vi "Add Property.vi"(6 "String?":bool, 7 "Include Empty?":bool, 9 "Value":string, 10 "Property Name":string, 11 "String In":string="{") -> (3 "String out":string)   [LabVIEW 2015, in "JSON.lvlib"]
doc: "This VI does not generate complete JSON!\n\nThis is a utility VI to help build partial JSON strings by adding a property to an object. If the property added isn't the first added to an object (the preceding character isn't '{') then it will prepend the property with the necessary comma. For this to work properly the first item being added should have \"{\" passed in as the partial JSON string and after all properties are added the JSON must be closed with \"}\"."
uses:
  JSON.lvlib
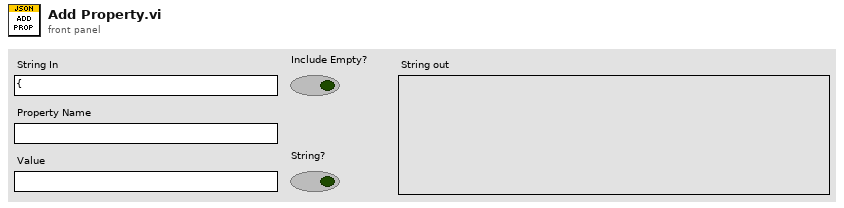
[diagram p1: front panel]
types:
  T1 = typedef "JSON.lvlib/JSON Item Type.ctl" = enum16{"unknown", "null", "Array", "Object", "String", "Number", "Boolean"}
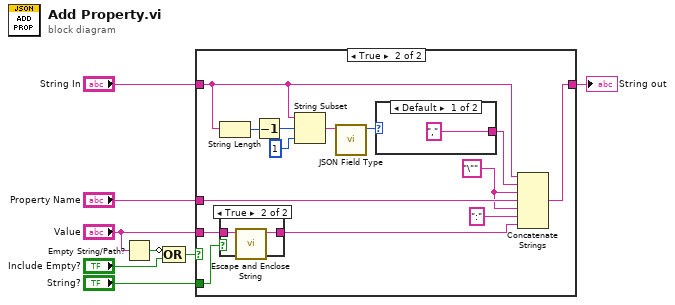
[diagram p0: block diagram]
diagram:
  n1 = Empty String/Path?(string/path="Value") -> (empty?=w8:bool)
  n2 = Compound Arithmetic op=OR(invert w8, "Include Empty?") -> (w6:bool)
  n3 = case shown="True" w6 {
    tunnel: "Value" -> [_ w19]
    tunnel: "Property Name" -> [_ w14]
    tunnel: "String In" -> [w9 w16]
    tunnel: [w9 w10] -> w2
    tunnel: "String?" -> [_ w18]
    frame False {
    }
    frame True {
      w11 = "\"" ("string")
      n4 = String Length(string=w16) -> (length=w23:i32)
      n5 = case shown="True" w18 {
        tunnel: w19 -> [w25 w27]
        tunnel: [w25 w26] -> w12
        frame False {
        }
        frame True {
          n6 = call "Escape and Enclose String.vi"("String"=w27) -> ("JSON String"=w26:string)  [unwired: 10 in]
        }
      }
      n7 = Decrement(x=w23) -> (x-1=w22:i32)
      n8 = String Subset(string=w16, offset (0)=w22, length (rest)=1 ("length (rest)")) -> (substring=w20:string)
      n9 = call "JSON Field Type.vi"("JSON String"=w20) -> ("JSON Item Type"=w17:T1)  [unwired: 10 in]
      n10 = case shown="Default" w17 {
        tunnel: ["," _] -> w15
        frame Default {
        }
        frame "Object" {
        }
      }
      n11 = Concatenate Strings(w16, w15, w11, w14, w11, ":" ("string"), w12) -> (w10:string)
    }
  }
  "String out" <- w2
